vi "HandleGroundPass.vi"(7 "InitState":T1, 8 "error in":errorcluster, 11 "Toggle?":bool) -> (0 "error out":errorcluster, 3 "State":T1)   [LabVIEW 2013]
uses:
  GroundPassWrapperStates.ctl
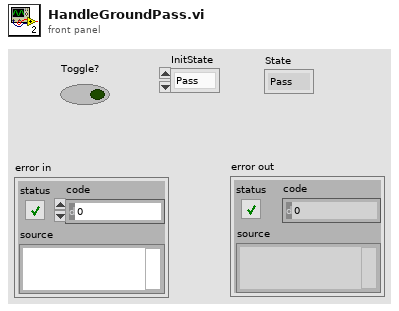
[diagram p1: front panel]
types:
  T1 = typedef "GroundPassWrapperStates.ctl" = enum16{"Pass", "Stop"}
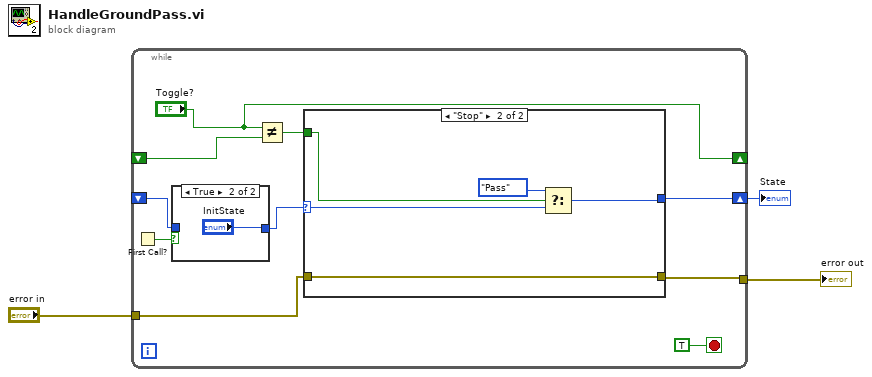
[diagram p0: block diagram]
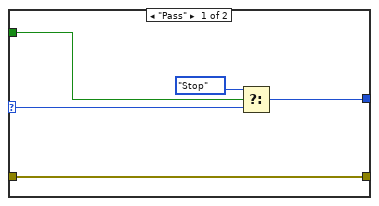
[diagram p3: hidden frame]
diagram:
  n1 = while {
    shift-right: ["Toggle?"] -> _
    shift-left: _ -> [w9]
    tunnel: "error in" -> [w11]
    tunnel: [w10] -> w2
    shift-right: [w5] -> w1
    shift-left: _ -> [w4]
    stop <- TRUE stop-if-true
    n2 = First Call?() -> (First Call?: T/F=w12:bool)
    n3 = case shown="True" w12 {
      tunnel: w4 -> [w14 _]
      tunnel: [w14 "InitState"] -> w6
      frame False {
      }
      frame True {
      }
    }
    n4 = Not Equal?(x="Toggle?", y=w9) -> (x != y?=w8:bool)
    n5 = case shown="\"Stop\"" w6 {
      selector: w6 -> [w17 w25]
      tunnel: w11 -> [w19 w22]
      tunnel: [w19 w22] -> w10
      tunnel: [w20 w23] -> w5
      tunnel: w8 -> [w18 w24]
      frame "Pass" {
        n6 = Select(t=GroundPassWrapperStates."Stop", s=w18, f=w17) -> (s? t:f=w20:T1)
      }
      frame "Stop" {
        n7 = Select(t=GroundPassWrapperStates."Pass", s=w24, f=w25) -> (s? t:f=w23:T1)
      }
    }
  }
  "error out" <- w2
  "State" <- w1
